vi "stopThread.vi"(0 "HGF_ThreadPool_Reference":refnum<class "HGF_Reference.lvclass">, 3 "timeout in ms (-1)":i32=-1, 5 "error in (no error)":errorcluster) -> (14 "dup HGF_ThreadPool_Reference":refnum<class "HGF_Reference.lvclass">, 17 "got object?":bool, 19 "error out":errorcluster)   [LabVIEW 2014, in "HGF_BaseClasses.lvlib" / "HGF_ThreadPool.lvclass"]
doc: "Use this VI to stop all threads of the referenced ThreadPool."
uses:
  HGF_ThreadPool.lvclass
  HGF_Reference/HGF_Reference.lvclass
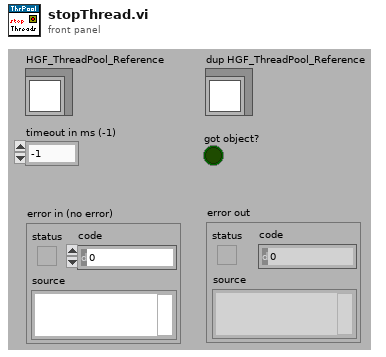
[diagram p1: front panel]
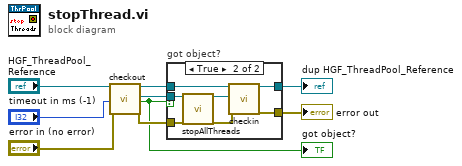
[diagram p0: block diagram]
diagram:
  n1 = call "checkout.vi"("HGF_ThreadPool_Reference"="HGF_ThreadPool_Reference", "timeout in ms (-1)"="timeout in ms (-1)", "error in (no error)"="error in (no error)") -> ("dup HGF_ThreadPool_Reference"=w5:refnum<class "HGF_Reference.lvclass">, "HGF_ThreadPool"=w8:refnum<class "HGF_ThreadPool.lvclass">, "got object?"=w2:bool, "error out"=w7:errorcluster)  [unwired: 13 out]
  "got object?" <- w2
  n2 = case "got object?" shown="True" w2 {
    tunnel: w8 -> [_ w18]
    tunnel: w7 -> [w10 w17]
    tunnel: w5 -> [w11 w14]
    tunnel: [w11 w13] -> w4
    tunnel: [w10 w12] -> w3
    frame False {
    }
    frame True {
      n3 = call "stopAllThreads.vi"("HGF_ThreadPool"=w18, "error in (no error)"=w17) -> ("dup HGF_ThreadPool"=w16:refnum<class "HGF_ThreadPool.lvclass">, "error out"=w15:errorcluster)  [unwired: 16 out]
      n4 = call "checkin.vi"("HGF_Reference"=w14, "Object"=w16, "error in (no error)"=w15) -> ("dup HGF_Reference"=w13:refnum<class "HGF_Reference.lvclass">, "error out"=w12:errorcluster)  [unwired: 1 in, 14 out]
    }
  }
  "error out" <- w3
  "dup HGF_ThreadPool_Reference" <- w4
